vi "3.vi"() -> ()   [LabVIEW 2017]
panel:
  out "添加的数组":dbl[][](array[numeric])
  out "数组":dbl[][](array[numeric])
  out "波形图":dbl[][](graph)
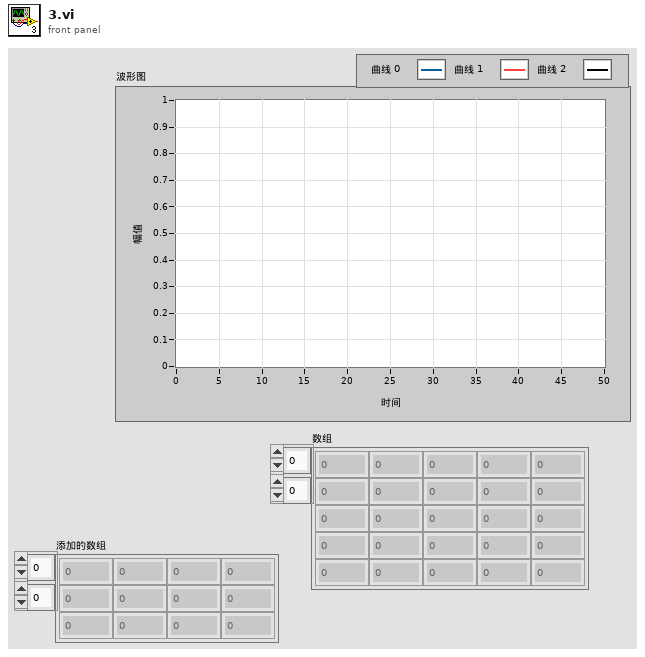
[diagram p1: front panel]
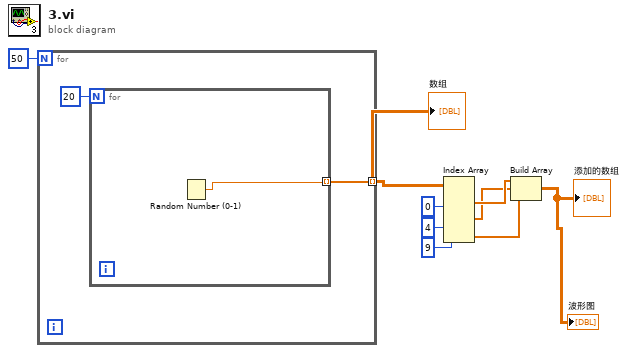
[diagram p0: block diagram]
diagram:
  n1 = for {
    N: 50 -> [_]
    tunnel: [w10] -> w8 mode=indexing
    n2 = for {
      N: 20 -> [_]
      tunnel: [w12] -> w10 mode=indexing
      n3 = Random Number (0-1)() -> (number: 0 to 1=w12:dbl)
    }
  }
  "数组" <- w8
  n4 = Index Array(array=w8, index (col) #1=0 ("禁用的索引 (列)"), index (col) #2=4 ("索引 (列)"), index (col) #3=9 ("索引 (列)")) -> (element #1=w4:dbl[], element #2=w3:dbl[], element #3=w2:dbl[])  [unwired: 3 in]
  n5 = Build Array(w4, w3, w2) -> (→"波形图" →"添加的数组":dbl[][])
